vi "Global 2.vi"() -> ()   [LabVIEW 2015]
panel:
  out "ŒREDNIE NAPEDY":T1
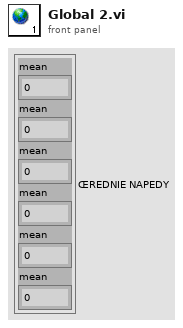
[diagram p1: front panel]
types:
  T1 = cluster{"mean":dbl, "mean":dbl, "mean":dbl, "mean":dbl, "mean":dbl, "mean":dbl}
diagram:
